vi "PLC Rotate Puck.vi"(11 "Rotate":T1={"Mode"=1, "PV Angle"=0.0, "SP_Angle"=0.0, "Rotate Angle"=0.0, "Timeout"=0.0, "Start"=FALSE, "Home"=FALSE} {"Rotate Angle" format="%.1f"; "SP_Angle" format="%.1f"; "PV Angle" format="%.2f"; "Mode" items=["Поворот"=1, "Качение"=2]}) -> (3 "appended array":u16[](array[numeric]))   [LabVIEW 2018, in "Drive.lvlib"]
uses:
  Drive.lvlib
  Rotation Control Type.ctl
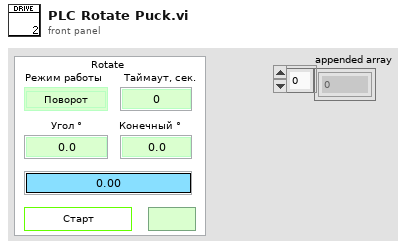
[diagram p1: front panel]
types:
  T1 = typedef "Drive.lvlib/Rotation Control Type.ctl" = cluster{"Mode":u16, "PV Angle":dbl, "SP_Angle":dbl, "Rotate Angle":dbl, "Timeout":dbl, "Start":bool, "Home":bool}
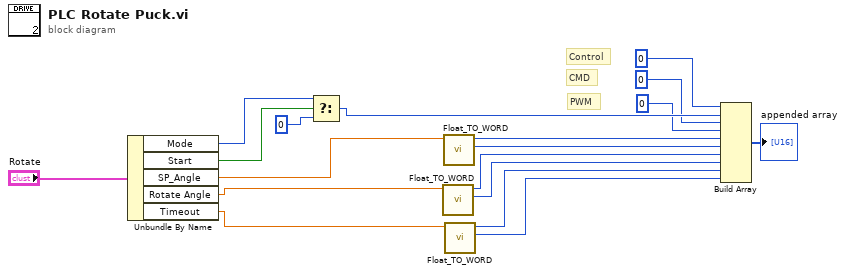
[diagram p0: block diagram]
diagram:
  # "CMD"
  # "PWM"
  # "Control"
  n1 = Unbundle By Name("Rotate") -> ("Mode"=w16:u16, "Start"=w17:bool, "SP_Angle"=w11:dbl, "Rotate Angle"=w10:dbl, "Timeout"=w9:dbl)
  n2 = Select(t=w16, s=w17, f=u16 0) -> (s? t:f=w13:u16)
  n3 = call "Float_TO_WORD.vi"("FLOAT"=w10) -> ("second_Word"=w5:u16, "first_Word"=w6:u16)  [unwired: 9 in]
  n4 = call "Float_TO_WORD.vi"("FLOAT"=w11) -> ("second_Word"=w7:u16, "first_Word"=w8:u16)  [unwired: 9 in]
  n5 = call "Float_TO_WORD.vi"("FLOAT"=w9) -> ("second_Word"=w3:u16, "first_Word"=w4:u16)  [unwired: 9 in]
  n6 = Build Array(u16 0 ("f"), w13, u16 0 ("f"), u16 0 ("f"), w8, w7, w6, w5, w4, w3) -> (→"appended array":u16[])
